vi "prompt_dialog.vi"(0 "Enable":bool=TRUE, 1 "caption":string, 2 "Display Style":u32, 5 "error in (no error)":errorcluster) -> (17 "Value":string, 18 "OK":bool, 19 "error out":errorcluster)   [LabVIEW 2010]
doc: "Displays a standard dialog box that prompts users to enter information, such as a user name and password.\n--------------------\n\nThis Express VI is configured as follows:\n\nMessage to Display to the User:\nThe inputs are: \nText Entry Box: Password"
panel:
  in  "Value":string caption="Enter the password for joe"
  in  "Cancel":bool
  in  "OK2":bool
  in  "OK1":bool
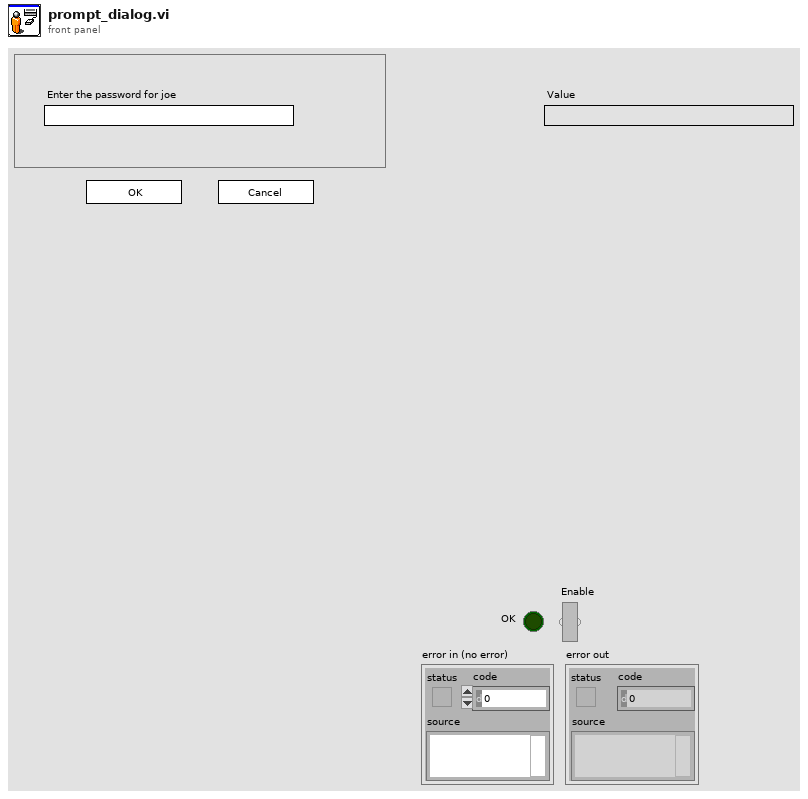
[diagram p1: front panel]
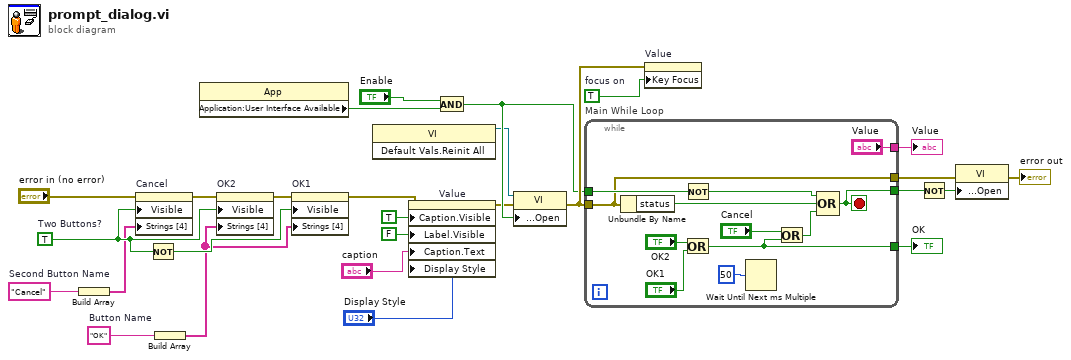
[diagram p0: block diagram]
diagram:
  w8 = TRUE  # focus on
  w19 = "Cancel"  # Second Button Name
  w17 = "OK"  # Button Name
  w27 = TRUE  # Two Buttons?
  n1 = Build Array(w19) -> (w20:string[])
  n2 = property on="Cancel" class="Bool"(error in="error in (no error)", "Visible"=w27, "Strings [4]"=w20) -> (error out=w24:errorcluster)  [unwired: 1 in, 1 out]
  n3 = Not(x=w27) -> (.not. x?=w25:bool)
  n4 = Build Array(w17) -> (w18:string[])
  n5 = property class="App"() -> ("Application:User Interface Available"=w10:bool)  [unwired: 2 in, 2 out]
  n6 = property on="OK2" class="Bool"(error in=w24, "Visible"=w27, "Strings [4]"=w18) -> (error out=w23:errorcluster)  [unwired: 1 in, 1 out]
  n7 = property on="OK1" class="Bool"(error in=w23, "Visible"=w25, "Strings [4]"=w18) -> (error out=w7:errorcluster)  [unwired: 1 in, 1 out]
  n8 = invoke class="VI" method="Default Vals.Reinit All"() -> (reference out=w9:refnum<vi>)  [unwired: 3 in, 2 out]
  n9 = property on="Value" class="Str"(error in=w7, "Caption.Visible"=TRUE, "Label.Visible"=FALSE, "Caption.Text"="caption", "Display Style"="Display Style") -> (error out=w6:errorcluster)  [unwired: 1 in, 1 out]
  n10 = And(x="Enable", y=w10) -> (x .and. y?=w11:bool)
  n11 = property class="VI"(reference=w9, error in=w6, "Front Panel Window:Open"=w11) -> (error out=w16:errorcluster)  [unwired: 1 out]
  n12 = while "Main While Loop" {
    tunnel: [w36] -> w26
    tunnel: w11 -> [w34]
    tunnel: [w32] -> w21
    tunnel: w16 -> [w31]
    tunnel: [w31] -> w14
    tunnel: ["Value"] -> w5
    stop <- w32 stop-if-true
    n13 = Unbundle By Name(w31) -> ("status"=w29:bool)
    n14 = Not(x=w34) -> (.not. x?=w33:bool)
    n15 = Or(x="OK2", y="OK1") -> (x .or. y?=w36:bool)
    n16 = Wait Until Next ms Multiple(millisecond multiple=u32 50) -> ()  [unwired: 1 out]
    n17 = Or(x="Cancel", y=w36) -> (x .or. y?=w30:bool)
    n18 = Compound Arithmetic op=OR(w33, w29, w30) -> (w32:bool)
  }
  "OK" <- w26
  "Value" <- w5
  n19 = property on="Value" class="Str"(error in=w16, "Key Focus"=w8) -> ()  [unwired: 1 in, 2 out]
  n20 = Not(x=w21) -> (.not. x?=w22:bool)
  n21 = property class="VI"(error in=w14, "Front Panel Window:Open"=w22) -> (error out=→"error out":errorcluster)  [unwired: 1 in, 1 out]
